vi "Is Concrete Class.vi"(0 "Path Group in":refnum<class "Path Group.lvclass">, 11 "error in (no error)":errorcluster) -> (4 "Path Group out":refnum<class "Path Group.lvclass">, 6 "Is Concrete Class?":bool=TRUE, 15 "error out":errorcluster)   [LabVIEW 2023, in "RFCalAndFixtureCharact.Common.lvlib" / "Path Group.lvclass"]
uses:
  Path Group.lvclass
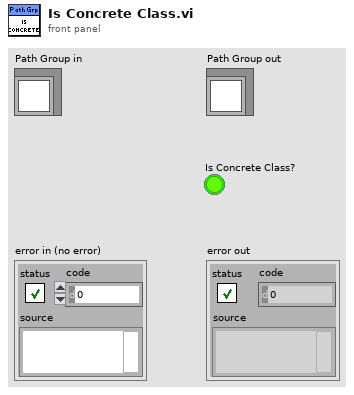
[diagram p1: front panel]
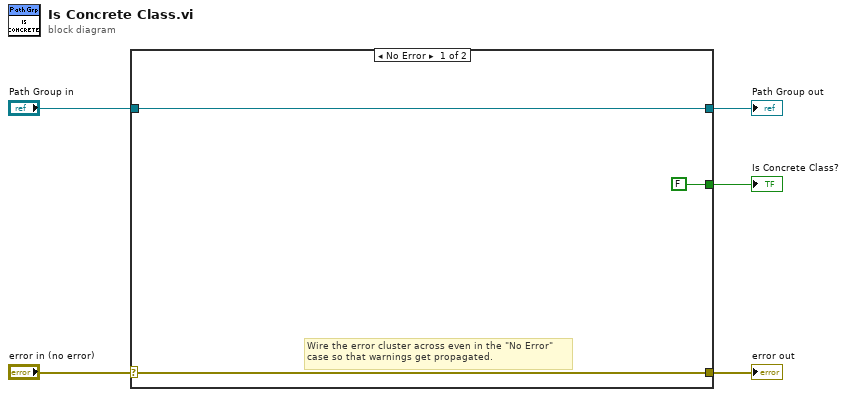
[diagram p0: block diagram]
diagram:
  n1 = case shown="No Error" "error in (no error)" {
    selector: "error in (no error)" -> [w7 w10]
    tunnel: [w7 w10] -> w4
    tunnel: [w8 w9] -> w2
    tunnel: "Path Group in" -> [w8 w9]
    tunnel: [FALSE ("Is Concrete Class?") _] -> w1
    frame No Error {
      # "Wire the error cluster across even in the \"No Error\"\ncase so that warnings get propagated."
    }
    frame Error {
    }
  }
  "error out" <- w4
  "Path Group out" <- w2
  "Is Concrete Class?" <- w1
